vi "executeOffensivePlay.vi"(8 "error in (no error)":errorcluster, 11 "Game in":refnum<class "Game.lvclass">) -> (0 "error out":errorcluster, 3 "Game out":refnum<class "Game.lvclass">)   [LabVIEW 2020, in "Game.lvclass"]
uses:
  Game.lvclass
  Utilities_class/Utilities.lvclass
  Team_class/OffensivePlay.ctl
  Game.lvclass/Game.ctl
  Team_class/Team.lvclass/Team.ctl
  Playbook_class/Playbook.lvclass/Playbook.ctl
  StopOffensivePlay_class/StopOffensivePlay.lvclass/StopOffensivePlay.ctl
  Robot_class/Robot.lvclass/Robot.ctl
  Robot_class/Read role.vi
  Playbook_class/Read offensive_plays.vi
  StopOffensivePlay_class/Read Roles.vi
  Read OffensiveTeam.vi
  Read FieldRef.vi
  Team_class/Read RobotRef.vi
  Team_class/Read OffensivePlay.vi
  Team_class/Write RobotRef.vi
  Write OffensiveTeam.vi
  Ally_class/Ally.lvclass
  C:/Users/Pedro/Dropbox/My PC (LAPTOP-06JBDO7V)/Documents/GitHub/SSL_AI/Team_class/Team.lvclass
  Playbook_class/Playbook.lvclass
  Field_class/Field.lvclass
  Robot_class/Robot.lvclass
  Play_class/Play.lvclass
  TestPlay_class/TestPlay.lvclass
  EnemyPossessionAtEnemyFieldPlay_class/EnemyPossessionAtEnemyFieldPlay.lvclass
  EnemyPossessionAtOurFieldPlay_class/EnemyPossessionAtOurFieldPlay.lvclass
  NormalGamePlay_class/NormalGamePlay.lvclass
  IndirectEnemyPlay_class/IndirectEnemyPlay.lvclass
  PrepareKickoffAllyPlay_class/PrepareKickoffAllyPlay.lvclass
  PrepareKickoffEnemyPlay_class/PrepareKickoffEnemyPlay.lvclass
  KickPenaltyAllyPlay_class/KickPenaltyAllyPlay.lvclass
  PreparePenaltyAllyPlay_class/PreparePenaltyAllyPlay.lvclass
  DirectEnemyPlay_class/DirectEnemyPlay.lvclass
  PreparePenaltyEnemyPlay_class/PreparePenaltyEnemyPlay.lvclass
  BallOutOfFieldPlay_class/BallOutOfFieldPlay.lvclass
  StopOffensivePlay_class/StopOffensivePlay.lvclass
  PassPlay_class/PassPlay.lvclass
  DirectKickPlay_class/DirectKickPlay.lvclass
  HaltPlay_class/HaltPlay.lvclass
  PreparePassPlay_class/PreparePassPlay.lvclass
  PassToStriker_class/PassToStriker.lvclass
  PassTo2ndStriker_class/PassTo2ndStriker.lvclass
  MarkerRole_class/MarkerRole.lvclass
  AttackerStopRole_class/AttackerStopRole.lvclass
  ShootRole_class/ShootRole.lvclass
  FollowAttackerRole_class/FollowAttackerRole.lvclass
  DefaultPsRole_class/DefaultPsRole.lvclass
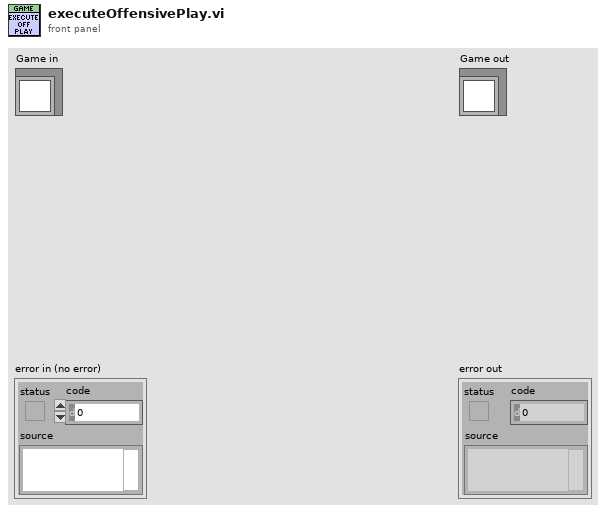
[diagram p1: front panel]
types:
  T1 = typedef "OffensivePlay.ctl" = enum16{"PreparePass", "PassToStriker", "BallOutOfField", "PassTo2ndStriker", "StopOffensive", "Prepare Penalty Enemy", "EnemyPossessionAtEnemyField", "EnemyPossesionAtOurField", "TestPlay", "PreparePenaltyAlly", "KickPenaltyAlly", "PrepareKickoffAlly", "PrepareKickoffEnemy", "IndirectEnemy", "DirectEnemy", "NormalGame", "DirectKick", "Pass", "Halt", "Timeout", "PassPlay", "PenaltyEnemy"}
  T2 = typedef "offensive_plays.ctl" = cluster{"Play":refnum<class "Play.lvclass">, "TestPlay":refnum<class "TestPlay.lvclass">, "EnemyPossessionAtEnemyFieldPlay":refnum<class "EnemyPossessionAtEnemyFieldPlay.lvclass">, "EnemyPossessionAtOurFieldPlay":refnum<class "EnemyPossessionAtOurFieldPlay.lvclass">, "NormalGamePlay":refnum<class "NormalGamePlay.lvclass">, "IndirectEnemyPlay":refnum<class "IndirectEnemyPlay.lvclass">, "PrepareKickoffAllyPlay":refnum<class "PrepareKickoffAllyPlay.lvclass">, "PrepareKickoffEnemyPlay":refnum<class "PrepareKickoffEnemyPlay.lvclass">, "KickPenaltyAllyPlay":refnum<class "KickPenaltyAllyPlay.lvclass">, "PreparePenaltyAllyPlay":refnum<class "PreparePenaltyAllyPlay.lvclass">, "DirectEnemyPlay":refnum<class "DirectEnemyPlay.lvclass">, "PreparePenaltyEnemyPlay":refnum<class "PreparePenaltyEnemyPlay.lvclass">, "BallOutOfFieldPlay":refnum<class "BallOutOfFieldPlay.lvclass">, "StopOffensivePlay":refnum<class "StopOffensivePlay.lvclass">, "PassPlay":refnum<class "PassPlay.lvclass">, "DirectKickPlay":refnum<class "DirectKickPlay.lvclass">, "HaltPlay":refnum<class "HaltPlay.lvclass">, "PreparePassPlay":refnum<class "PreparePassPlay.lvclass">, "PassToStriker":refnum<class "PassToStriker.lvclass">, "PassTo2ndStriker":refnum<class "PassTo2ndStriker.lvclass">}
  T3 = typedef "roles.ctl" = enum16{"PenaltyDefense", "DefaultPs", "PreparePassReceiver", "PassObserver", "Timeout", "Goto", "ZigZag", "None", "BallOutOfField", "DefenderArea", "Duelist", "AttackerStop", "FollowAttacker", "KeeperRole", "KickPenalty", "AttackerAimGoal", "AttackerBlock", "Marker", "Halt", "Shoot", "PassKicker", "PassReceiver", "TestRole", "PenaltyAttacker"}
  T4 = cluster{"MarkerRole":refnum<class "MarkerRole.lvclass">, "AttackerStopRole":refnum<class "AttackerStopRole.lvclass">}
  T5 = cluster{"ShootRole":refnum<class "ShootRole.lvclass">, "FollowAttackerRole":refnum<class "FollowAttackerRole.lvclass">, "DefaultPsRole":refnum<class "DefaultPsRole.lvclass">}
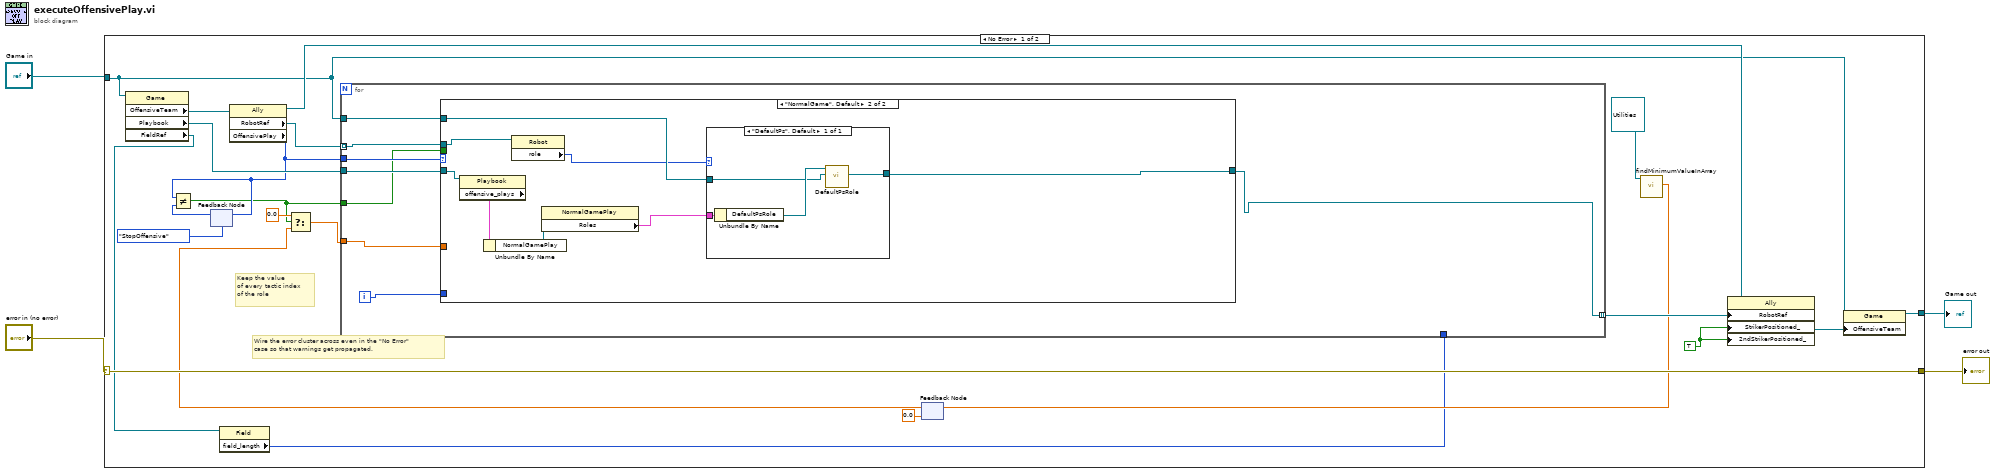
[diagram p0: block diagram]
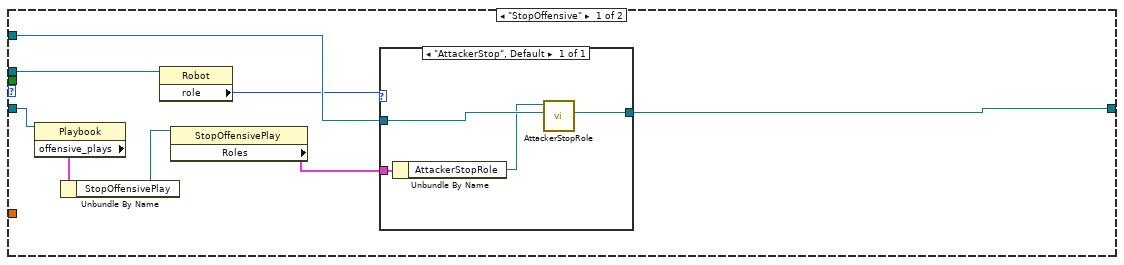
[diagram p2: hidden frame]
diagram:
  n1 = case shown="No Error" "error in (no error)" {
    selector: "error in (no error)" -> [w26 w60]
    tunnel: [w26 w60] -> w1
    tunnel: [w20 w59] -> w2
    tunnel: "Game in" -> [w5 w59]
    frame No Error {
      w9 = TRUE
      # "Keep the value\nof every tactic index\nof the role"
      # "Wire the error cluster across even in the \"No Error\"\ncase so that warnings get propagated."
      n2 = property class="Game"(reference=w5) -> ("OffensiveTeam"=w25:refnum<class "Ally.lvclass">, "Playbook"=w23:refnum<class "Playbook.lvclass">, "FieldRef"=w7:refnum<class "Field.lvclass">)  [unwired: 1 in, 2 out]
      n3 = feedback #1(OffensivePlay."StopOffensive" ("OffensivePlay")) -> (w15:T1)
      n4 = property class="Field"(reference=w7) -> ("field_length"=w6:i32)  [unwired: 1 in, 2 out]
      n5 = property class="Ally"(reference=w25) -> (reference out=w22:refnum<class "Ally.lvclass">, "RobotRef"=w24:refnum<class "Robot.lvclass">[], "OffensivePlay"=w16:T1)  [unwired: 1 in, 1 out]
      n6 = Not Equal?(x=w16, y=w15) -> (x != y?=w11:bool)
      n7 = feedback-in #1(w16) -> ()
      n8 = feedback #2(0.0 ("minimum")) -> (w13:dbl)
      n9 = Select(t=0.0, s=w11, f=w13) -> (s? t:f=w8:dbl)
      n10 = for {
        tunnel: w24 -> [w30] mode=indexing
        tunnel: w16 -> [w34]
        tunnel: w23 -> [w33]
        tunnel: w5 -> [w32]
        tunnel: [w27] -> w21 mode=indexing
        tunnel: w11 -> [w31]
        tunnel: w8 -> [w29]
        tunnel: w6 -> [_]
        i -> [w28]
        n11 = case shown="\"NormalGame\", Default" w34 {
          tunnel: w33 -> [w42 w54]
          tunnel: w32 -> [w38 w50]
          tunnel: [w37 w49] -> w27
          tunnel: w29 -> [_ _]
          tunnel: w31 -> [_ _]
          tunnel: w30 -> [w35 w48]
          tunnel: w28 -> [_ _]
          frame "StopOffensive" {
            n12 = property class="Playbook"(reference=w42) -> ("offensive_plays"=w41:T2)  [unwired: 1 in, 2 out]
            n13 = Unbundle By Name(w41) -> ("StopOffensivePlay"=w40:refnum<class "StopOffensivePlay.lvclass">)
            n14 = property class="Robot"(reference=w35) -> ("role"=w36:T3)  [unwired: 1 in, 2 out]
            n15 = property class="StopOffensivePlay"(reference=w40) -> ("Roles"=w39:T4)  [unwired: 1 in, 2 out]
            n16 = case shown="\"AttackerStop\", Default" w36 {
              tunnel: w39 -> [w46]
              tunnel: w38 -> [w45]
              tunnel: [w44] -> w37
              frame "AttackerStop", Default {
                n17 = Unbundle By Name(w46) -> ("AttackerStopRole"=w43:refnum<class "AttackerStopRole.lvclass">)
                n18 = call-dynamic "AttackerStopRole.vi"("Game in"=w45, "AttackerStopRole in"=w43) -> ("Robot out"=w44:refnum<class "Robot.lvclass">)  [unwired: 6 in, 3 out]
              }
            }
          }
          frame "NormalGame", Default {
            n19 = property class="Playbook"(reference=w54) -> ("offensive_plays"=w53:T2)  [unwired: 1 in, 2 out]
            n20 = Unbundle By Name(w53) -> ("NormalGamePlay"=w52:refnum<class "NormalGamePlay.lvclass">)
            n21 = property class="Robot"(reference=w48) -> ("role"=w47:T3)  [unwired: 1 in, 2 out]
            n22 = property class="NormalGamePlay"(reference=w52) -> ("Roles"=w51:T5)  [unwired: 1 in, 2 out]
            n23 = case shown="\"DefaultPs\", Default" w47 {
              tunnel: w51 -> [w58]
              tunnel: w50 -> [w56]
              tunnel: [w55] -> w49
              frame "DefaultPs", Default {
                n24 = Unbundle By Name(w58) -> ("DefaultPsRole"=w57:refnum<class "DefaultPsRole.lvclass">)
                n25 = call "DefaultPsRole.vi"("Game in"=w56, "DefaultPsRole in"=w57) -> ("Robot out"=w55:refnum<class "Robot.lvclass">)  [unwired: 7 in, 1 out]
              }
            }
          }
        }
      }
      n26 = call-dynamic "findMinimumValueInArray.vi"("Utilities in"=refnum<class "Utilities.lvclass"> refnum) -> ("minimum"=w17:dbl)  [unwired: 8 in, 2 out]
      n27 = feedback-in #2(w17) -> ()
      n28 = property class="Ally"(reference=w22, "RobotRef"=w21, "StrikerPositioned_"=w9, "2ndStrikerPositioned_"=w9) -> (reference out=w19:refnum<class "Ally.lvclass">)  [unwired: 1 in, 1 out]
      n29 = property class="Game"(reference=w5, "OffensiveTeam"=w19) -> (reference out=w20:refnum<class "Game.lvclass">)  [unwired: 1 in, 1 out]
    }
    frame Error {
    }
  }
  "error out" <- w1
  "Game out" <- w2
